vi "RemotelyFireUpQT.vi"(3 "Path":path=path "/Chris/new Chris/Projects/QT FAT-CIN prj/FatCIN/SamplesFiles/Sample.mov") -> ()   [LabVIEW 2010]
panel:
  out "Movie setting":string
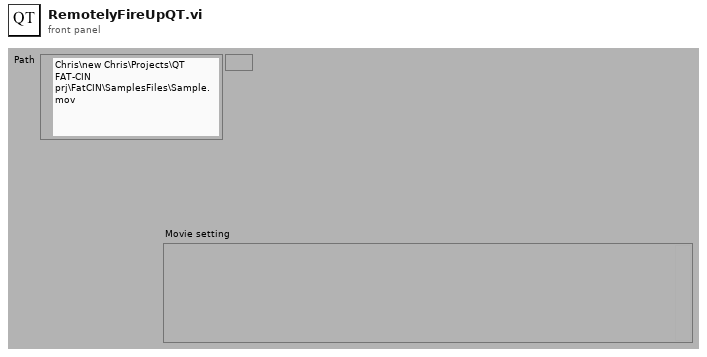
[diagram p1: front panel]
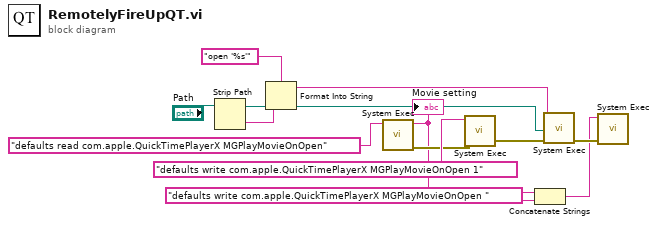
[diagram p0: block diagram]
diagram:
  n1 = Strip Path(path="Path") -> (stripped path=w11:path, name=w10:string)
  n2 = Format Into String(format string="open '%s'", w10) -> (resulting string=w9:string)  [unwired: 2 in, 1 out]
  n3 = call <vilib>:"System Exec.vi"("command line"="defaults read com.apple.QuickTimePlayerX MGPlayMovieOnOpen" ("format string")) -> ("error out"=w6:errorcluster, "standard output"=w4:string)  [unwired: 7 in, 2 out]
  "Movie setting" <- w4
  n4 = call <vilib>:"System Exec.vi"("error in (no error)"=w6, "command line"="defaults write com.apple.QuickTimePlayerX MGPlayMovieOnOpen 1" ("format string")) -> ("error out"=w3:errorcluster)  [unwired: 6 in, 3 out]
  n5 = Concatenate Strings("defaults write com.apple.QuickTimePlayerX MGPlayMovieOnOpen " ("format string"), w4) -> (w1:string)
  n6 = call <vilib>:"System Exec.vi"("error in (no error)"=w3, "working directory"=w11, "command line"=w9) -> ("error out"=w2:errorcluster)  [unwired: 5 in, 3 out]
  n7 = call <vilib>:"System Exec.vi"("error in (no error)"=w2, "command line"=w1) -> ()  [unwired: 6 in, 4 out]
